vi "BNC555.evt call Config Sys (To) Mode.vi"(0 "i ref in":refnum<vi>, 2 "Generator Instance":string="N/A", 3 "Mode":T1(ring), 5 "error in (no error)":errorcluster, 7 "Burst # (10)":u32=10, 9 "DC On (10)":u32=10, 11 "DC Off (10)":u32=10) -> (14 "i ref out":refnum<vi>, 19 "error out":errorcluster)   [LabVIEW 2014, in "BNC555.lvlib"]
doc: "This VI sends a simple event call to the wired BNC555."
uses:
  BNC555.lvlib
  CSCore/CSSystem/CoreLib/CoreLib.int 2 byte array.vi
  CSCore/CSSystem/CoreLib/CoreLib.short 2 byte array.vi
  CSCore/CSSystem/CoreLib/CoreLib.lvlib
  CSCore/BaseProcess/BaseProcess.lvlib
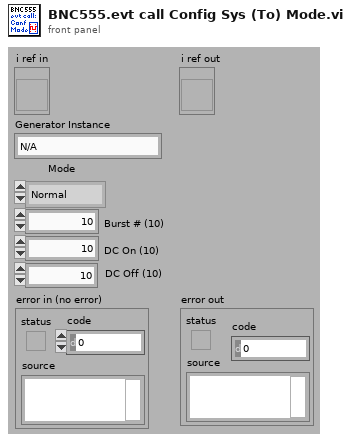
[diagram p1: front panel]
types:
  T1 = enum16{"Normal", "Single", "Burst", "Duty Cycle"}
  T2 = typedef "CoreDefs.rawDataType.ctl" = i8[]
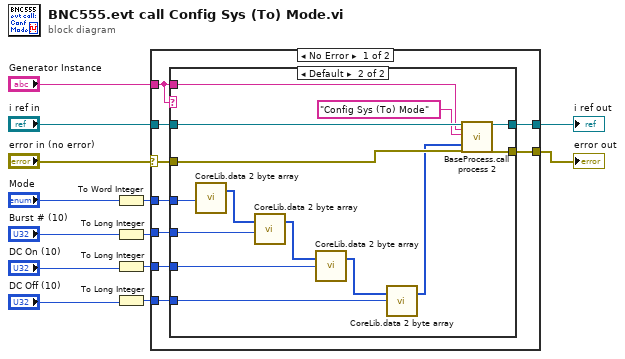
[diagram p0: block diagram]
diagram:
  n1 = To Word Integer(number="Mode") -> (16bit integer=w8:i16)
  n2 = To Long Integer(number="Burst # (10)") -> (32bit integer=w1:i32)
  n3 = To Long Integer(number="DC On (10)") -> (32bit integer=w7:i32)
  n4 = To Long Integer(number="DC Off (10)") -> (32bit integer=w6:i32)
  n5 = case shown="No Error" "error in (no error)" {
    selector: "error in (no error)" -> [w19 w39]
    tunnel: [w22 w40] -> w12
    tunnel: [w21 w39] -> w11
    tunnel: "i ref in" -> [w20 w40]
    tunnel: "Generator Instance" -> [w18 _]
    tunnel: w8 -> [w17 _]
    tunnel: w1 -> [w16 _]
    tunnel: w7 -> [w15 _]
    tunnel: w6 -> [w14 _]
    frame No Error {
      n6 = case shown="Default" w18 {
        tunnel: [w24 w38] -> w22
        tunnel: [w23 w37] -> w21
        tunnel: w20 -> [w24 w36]
        tunnel: w18 -> [_ w35]
        tunnel: w19 -> [w23 w33]
        tunnel: w17 -> [_ w28]
        tunnel: w16 -> [_ w27]
        tunnel: w15 -> [_ w26]
        tunnel: w14 -> [_ w25]
        frame "N/A" {
        }
        frame Default {
          n7 = call-poly "CoreLib.data 2 byte array.vi"("i16"=w28) -> ("byteArray out"=w32:T2)  [unwired: 18 in]
          n8 = call-poly "CoreLib.data 2 byte array.vi"("byteArray"=w32, "i32"=w27) -> ("byteArray out"=w31:T2)  [unwired: 17 in]
          n9 = call-poly "CoreLib.data 2 byte array.vi"("byteArray"=w31, "i32"=w26) -> ("byteArray out"=w30:T2)  [unwired: 17 in]
          n10 = call-poly "CoreLib.data 2 byte array.vi"("byteArray"=w30, "i32"=w25) -> ("byteArray out"=w29:T2)  [unwired: 17 in]
          n11 = call "BaseProcess.call process 2.vi"("i ref in"=w36, "Object"=w35, "Selector"="Config Sys (To) Mode", "Data"=w29, "error in (no error)"=w33) -> ("i ref out"=w38:refnum<vi>, "error out"=w37:errorcluster)  [unwired: 13 in]
        }
      }
    }
    frame Error {
    }
  }
  "error out" <- w11
  "i ref out" <- w12
